vi "Remove Subscriber.vi"(8 "error in (no error)":errorcluster, 10 "Publisher to Remove":string, 11 "CIF_Fifo_U8 in":refnum<class "CIF_Fifo_U8_Multi.lvclass">) -> (0 "error out":errorcluster, 3 "CIF_Fifo_U8 out":refnum<class "CIF_Fifo_U8_Multi.lvclass">)   [LabVIEW 2021, in "CIF_Fifo_U8_Multi.lvclass"]
uses:
  CIF_Fifo_U8_Multi.lvclass
  CIF_Fifo_U8_Multi.lvclass/CIF_Fifo_U8_Multi.ctl
  CIFChannels/CIFChannels.lvclass/CIFChannels.ctl
  ChannelCommon/typedef/Errors.ctl
  CIFChannels/Accessors/Read Name.vi
  <vilib>/CIF Foundation/CIF Utilities/Errors/Append Error Location.vi
  FIFO_U8/CIF_NIChn_Fifo_U8.lvclass
  D:/dev/Packages/CIF_Channels_Core/src/CIFChannels/CIFChannels.lvclass
  ChannelCommon/ChannelCommon.lvlib
  CIFChannels/Typedef/Channel State.ctl
  CIFChannels/CIFChannels.lvclass
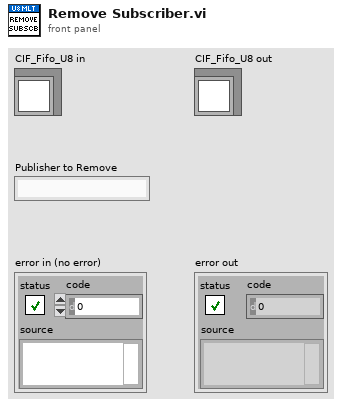
[diagram p1: front panel]
types:
  T1 = typedef "CIFChannels.lvclass/Channel State.ctl" = enum16{"Creating", "Disconnected", "Connecting", "Connected", "Destroyed"}
  T2 = typedef "ChannelCommon.lvlib/Errors.ctl" = enum16{"gRPC Server Not Found", "Duplicate Channel", "Missing Channel", "Incorrect Type", "Flatten Error", "Unflatten Data", "Channel Length", "Plugin Connection", "gRPC Server Connection", "FIFO Unflatten", "Required Override", "Remove Not Found", "Not Supported"}
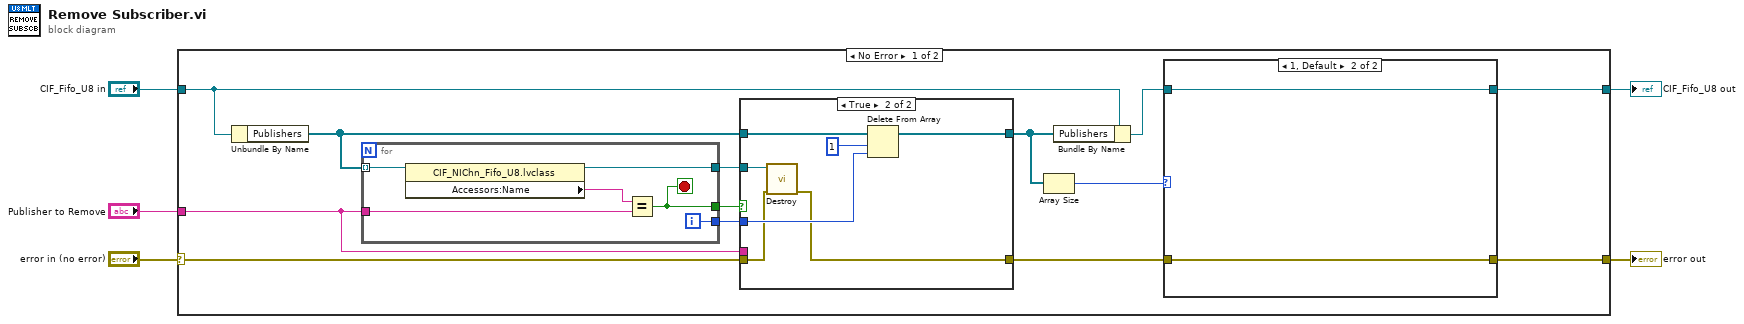
[diagram p0: block diagram]
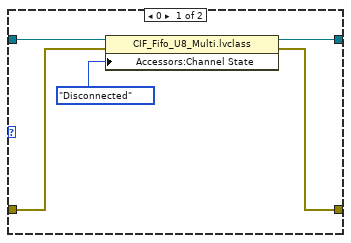
[diagram p2: hidden frame]
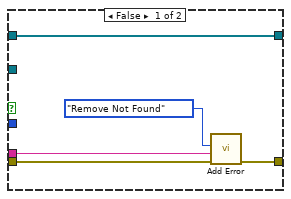
[diagram p3: hidden frame]
diagram:
  n1 = case shown="No Error" "error in (no error)" {
    selector: "error in (no error)" -> [w13 w45]
    tunnel: [w6 w45] -> w4
    tunnel: [w8 w44] -> w2
    tunnel: "CIF_Fifo_U8 in" -> [w18 w44]
    tunnel: "Publisher to Remove" -> [w12 _]
    frame No Error {
      n2 = Unbundle By Name(w18) -> ("Publishers"=w14:refnum<class "CIF_NIChn_Fifo_U8.lvclass">[])
      n3 = for {
        tunnel: w14 -> [w43] mode=indexing
        tunnel: w12 -> [w41]
        tunnel: [w40] -> w17
        tunnel: [w39] -> w16
        tunnel: [w38] -> w15
        i -> [w38]
        stop <- w39 stop-if-true
        n4 = property class="CIF_NIChn_Fifo_U8.lvclass"(reference=w43) -> (reference out=w40:refnum<class "CIF_NIChn_Fifo_U8.lvclass">, "Accessors:Name"=w42:string)  [unwired: 1 in, 1 out]
        n5 = Equal?(x=w42, y=w41) -> (x = y?=w39:bool)
      }
      n6 = case shown="True" w16 {
        tunnel: w14 -> [w30 w37]
        tunnel: w17 -> [_ w36]
        tunnel: w15 -> [_ w35]
        tunnel: w13 -> [w29 w33]
        tunnel: [w28 w32] -> w7
        tunnel: [w30 w31] -> w11
        tunnel: w12 -> [w26 _]
        frame False {
          n7 = call "Add Error.vi"("error in (no error)"=w29, "String to Append"=w26, "Error"=Errors."Remove Not Found") -> ("error out"=w28:errorcluster)  [unwired: 8 in]
        }
        frame True {
          n8 = call-dynamic "Destroy.vi"("error in (no error)"=w33, "CIFFIFO in"=w36) -> ("error out"=w32:errorcluster)  [unwired: 8 in, 1 out]
          n9 = Delete From Array(array=w37, length=1, index=w35) -> (array with subset deleted=w31:refnum<class "CIF_NIChn_Fifo_U8.lvclass">[])  [unwired: 1 out]
        }
      }
      n10 = Array Size(array=w11) -> (size(s)=w10:i32)
      n11 = Bundle By Name(cluster=w18, "Publishers"=w11) -> (w9:refnum<class "CIF_Fifo_U8_Multi.lvclass">)
      n12 = case shown="1, Default" w10 {
        tunnel: w9 -> [w23 w25]
        tunnel: [w20 w25] -> w8
        tunnel: w7 -> [w21 w24]
        tunnel: [w19 w24] -> w6
        frame 0 {
          n13 = property class="CIF_Fifo_U8_Multi.lvclass"(reference=w23, error in=w21, "Accessors:Channel State"=Channel_State."Disconnected" ("Channel State")) -> (reference out=w20:refnum<class "CIF_Fifo_U8_Multi.lvclass">, error out=w19:errorcluster)
        }
        frame 1, Default {
        }
      }
    }
    frame Error {
    }
  }
  "error out" <- w4
  "CIF_Fifo_U8 out" <- w2
